vi "Experiment_start_tasks.vi"(0 "Experiment (in)":refnum<class "Experiment.lvclass">, 5 "error in":errorcluster) -> (14 "Experiment":refnum<class "Experiment.lvclass">, 19 "error out":errorcluster)   [LabVIEW 2013, in "Experiment.lvclass"]
uses:
  Experiment.lvclass
  Experiment.lvclass/Experiment.ctl
  Counter/Counter.lvclass
  Analog_output/Analog_Output.lvclass
  DAQmx_pulse_out/DAQmx_pulse_out.lvclass
  HSDIO/HSDIO.lvclass
  ExperimentVariables/ExperimentVariables.lvclass
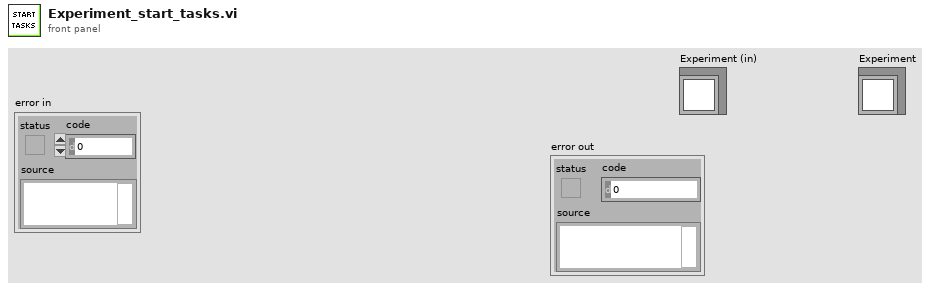
[diagram p1: front panel]
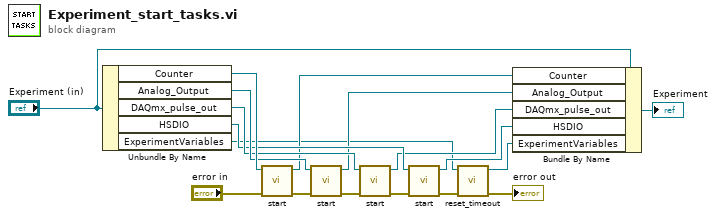
[diagram p0: block diagram]
diagram:
  n1 = Unbundle By Name("Experiment (in)") -> ("Counter"=w14:refnum<class "Counter.lvclass">, "Analog_Output"=w13:refnum<class "Analog_Output.lvclass">, "DAQmx_pulse_out"=w12:refnum<class "DAQmx_pulse_out.lvclass">, "HSDIO"=w11:refnum<class "HSDIO.lvclass">, "ExperimentVariables"=w4:refnum<class "ExperimentVariables.lvclass">)
  n2 = call-dynamic "start.vi"("error in (no error)"="error in", "Counter in"=w14) -> ("error out"=w17:errorcluster, "Counter out"=w9:refnum<class "Counter.lvclass">)  [unwired: 8 in]
  n3 = call-dynamic "start.vi"("error in (no error)"=w17, "Analog_Output in"=w13) -> ("error out"=w16:errorcluster, "Analog_Output out"=w8:refnum<class "Analog_Output.lvclass">)  [unwired: 8 in]
  n4 = call-dynamic "start.vi"("error in (no error)"=w16, "DAQmx_pulse_out in"=w12) -> ("error out"=w15:errorcluster, "DAQmx_pulse_out out"=w7:refnum<class "DAQmx_pulse_out.lvclass">)  [unwired: 8 in]
  n5 = call-dynamic "start.vi"("error in (no error)"=w15, "HSDIO in"=w11) -> ("error out"=w3:errorcluster, "HSDIO out"=w6:refnum<class "HSDIO.lvclass">)  [unwired: 8 in]
  n6 = call-dynamic "reset_timeout.vi"("error in (no error)"=w3, "ExperimentVariables in"=w4) -> ("error out"=→"error out":errorcluster, "ExperimentVariables out"=w2:refnum<class "ExperimentVariables.lvclass">)  [unwired: 8 in]
  n7 = Bundle By Name(cluster="Experiment (in)", "Counter"=w9, "Analog_Output"=w8, "DAQmx_pulse_out"=w7, "HSDIO"=w6, "ExperimentVariables"=w2) -> (→"Experiment":refnum<class "Experiment.lvclass">)
